vi "Initialize Front Panel.vi"(8 "error in (no error)":errorcluster, 11 "QuadViewManager in":refnum<class "QuadViewManager.lvclass">) -> (0 "error out":errorcluster, 3 "QuadViewManager out":refnum<class "QuadViewManager.lvclass">)   [LabVIEW 2015, in "QuadViewManager.lvlib" / "QuadViewManager.lvclass"]
doc: "<License>\nCopyright © 2017 Composed Systems, LLC | All rights reserved\nwww.composed.io\n\nAuthor: Ethan Stern <ethan.stern@composed.io>\n\nThis software is provided \"AS IS\" WITHOUT WARRANTIES, either express or implied, AND IS FOR EDUCATIONAL PURPOSES ONLY.\n</License>"
uses:
  QuadViewManager.lvclass
  Framework/IViewManager/IViewManager/IViewManager.lvclass/IViewManager.ctl
  QuadViewManager.lvclass/QuadViewManager.ctl
  Framework/IViewable/IViewable Messages/Insert Front Panel Msg/Insert Front Panel Msg.lvclass/Insert Front Panel Msg.ctl
  <vilib>/ActorFramework/Message Enqueuer/Message Enqueuer.lvclass/Message Enqueuer.ctl
  <vilib>/ActorFramework/Message Enqueuer/Enqueue.vi
  <vilib>/ActorFramework/Message Priority Queue/Priority Enqueue.vi
  Framework/IViewManager/IViewManager/IViewManager.lvclass
  Framework/IViewable/IViewable Messages/Insert Front Panel Msg/Insert Front Panel Msg.lvclass
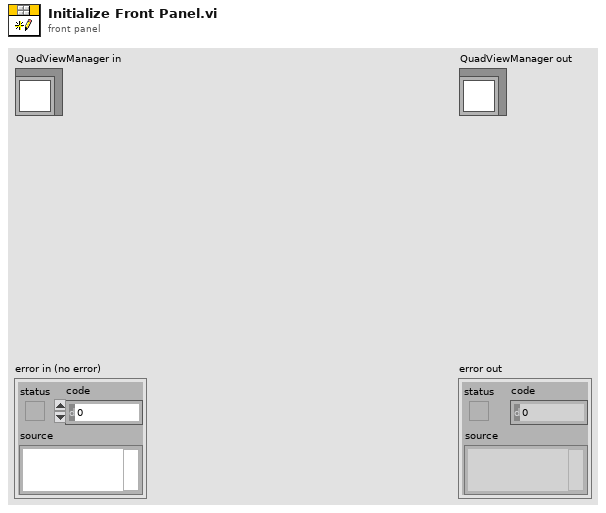
[diagram p1: front panel]
types:
  T1 = typedef "IViewable.lvlib/ProtectedSubpanel.lvclass/Protected Subpanel Reference.ctl" = refnum<data-value>
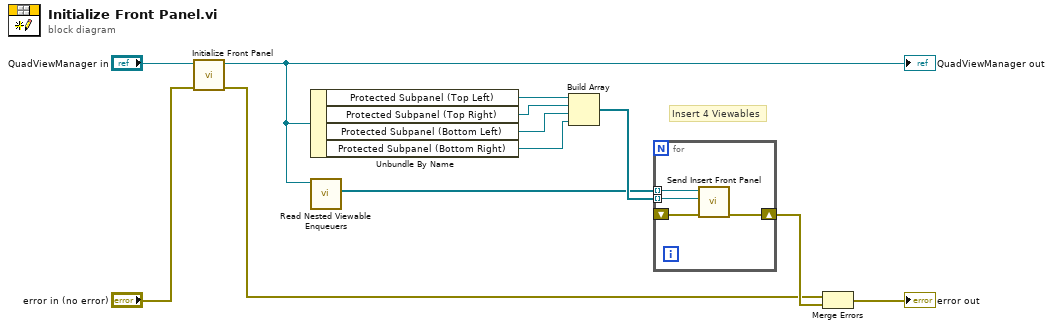
[diagram p0: block diagram]
diagram:
  # "Insert 4 Viewables"
  n1 = call-parent "Initialize Front Panel.vi"("error in (no error)"="error in (no error)", "IViewable in"="QuadViewManager in") -> ("error out"=w2:errorcluster, "IViewable out"=w3:refnum<class "QuadViewManager.lvclass">)  [unwired: 8 in]
  "QuadViewManager out" <- w3
  n2 = Unbundle By Name(w3) -> ("Protected Subpanel (Top Left)"=w10:T1, "Protected Subpanel (Top Right)"=w7:T1, "Protected Subpanel (Bottom Left)"=w8:T1, "Protected Subpanel (Bottom Right)"=w9:T1)
  n3 = call "Read Nested Viewable Enqueuers.vi"("IViewManager in"=w3) -> ("Nested Viewable Enqueuers"=w4:refnum<class "Message Enqueuer.lvclass">[])  [unwired: 9 in, 1 out]
  n4 = Build Array(w10, w7, w8, w9) -> (w6:T1[])
  n5 = for {
    tunnel: w6 -> [w16] mode=indexing
    shift-right: [w15] -> w5
    shift-left: _ -> [w14]
    tunnel: w4 -> [w13] mode=indexing
    n6 = call "Send Insert Front Panel.vi"("error in (no error)"=w14, "Protected Subpanel"=w16, "Message Enqueuer"=w13) -> ("error out"=w15:errorcluster)  [unwired: 7 in, 1 out]
  }
  n7 = Merge Errors(w2, w5) -> (→"error out":errorcluster)
